vi "Gate Valve Open_Closed.vi"(6 "data":u32[](array[numeric]), 7 "error in":errorcluster, 8 "G.V. Open?":bool, 9 "y":dbl, 10 "x":dbl) -> (0 "error out":errorcluster, 1 "Boolean":bool, 3 "String":string)   [LabVIEW 2013]
uses:
  <vilib>/DAQmx/write.llb/DAQmx Write.vi
  <vilib>/DAQmx/write.llb/DAQmx Write (Digital 1D U32 NChan 1Samp).vi
  <vilib>/DAQmx/miscellaneous.llb/DAQmx Fill In Error Info.vi
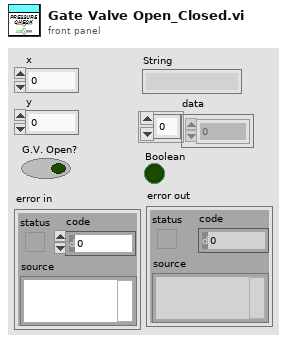
[diagram p1: front panel]
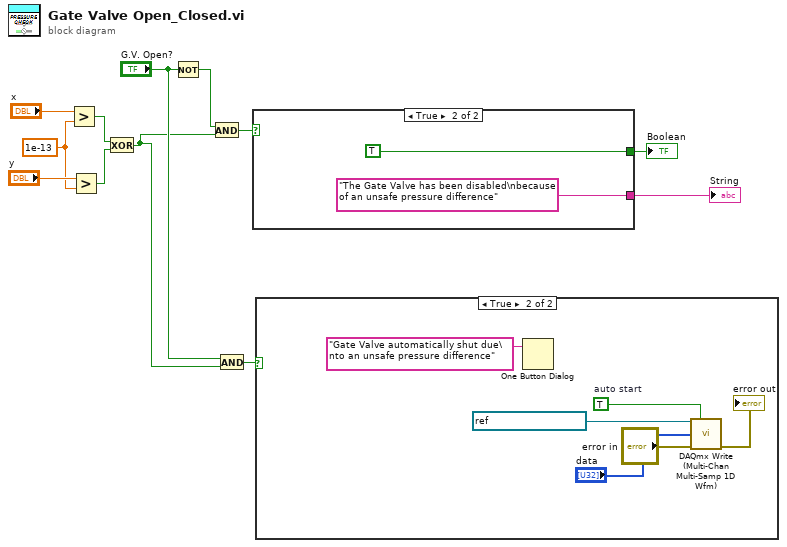
[diagram p0: block diagram]
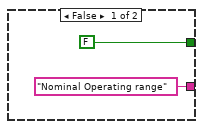
[diagram p3: hidden frame]
diagram:
  w8 = 1e-13 ("y")
  n1 = Greater?(x="x", y=w8) -> (0:w7:bool)
  n2 = Greater?(x="y", y=w8) -> (0:w6:bool)
  n3 = Exclusive Or(1:w6, 2:w7) -> (0:w1:bool)
  n4 = Not(x="G.V. Open?") -> (.not. x?=w11:bool)
  n5 = And(x=w11, y=w1) -> (x .and. y?=w12:bool)
  n6 = And(x="G.V. Open?", y=w1) -> (x .and. y?=w3:bool)
  n7 = case shown="True" w12 {
    tunnel: ["Nominal Operating range" "The Gate Valve has been disabled\nbecause of an unsafe pressure difference"] -> w5
    tunnel: [FALSE TRUE] -> w4
    frame False {
    }
    frame True {
    }
  }
  "String" <- w5
  "Boolean" <- w4
  n8 = case shown="True" w3 {
    frame False {
    }
    frame True {
      w22 = TRUE  # auto start
      n9 = One Button Dialog(message="Gate Valve automatically shut due\nto an unsafe pressure difference") -> ()  [unwired: 1 in, 1 out]
      n10 = call-poly "DAQmx Write (Multi-Chan Multi-Samp 1D Wfm).vi"("task/channels in"=refnum<k21> "DAQ Assistant_2" ("task in"), "auto start"=w22, "data"="data", "error in"="error in") -> ("error out"=→"error out":errorcluster)  [unwired: 9 in, 2 out]
    }
  }
